vi "Rescript.vi"() -> ()   [LabVIEW 2020]
uses:
  _Rescript/_Rescript/_Rescript.lvclass
  _Shared/_Shared.lvlib
  _Shared/Name Specs/Name Specs.lvclass
  _Shared/Tree/Tree.lvlib
panel:
  out "Target":string
  in  "Tree":string(tree)
  in  "OK":bool
  # "Disclaimer: Please consider committing changes before AND after this action."
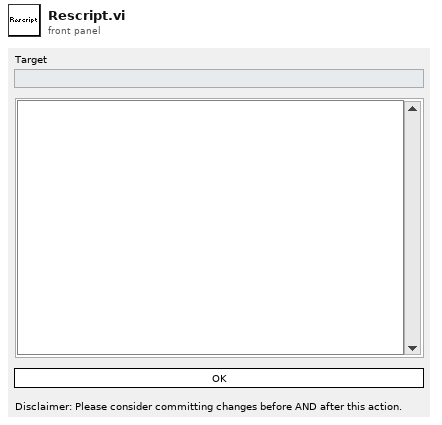
[diagram p1: front panel]
types:
  T1 = enum32{"Invalid", "Standard", "Closed", "Hidden", "Minimized", "Maximized"}
  T2 = typedef "_Shared.lvlib/Type Name Library File Path.ctl" = map{T3, T4}
  T3 = typedef "_Shared.lvlib/Type.ctl" = enum16{"Actor", "Msg"}
  T4 = typedef "_Shared.lvlib/Name Library File Path.ctl" = map{string, path}
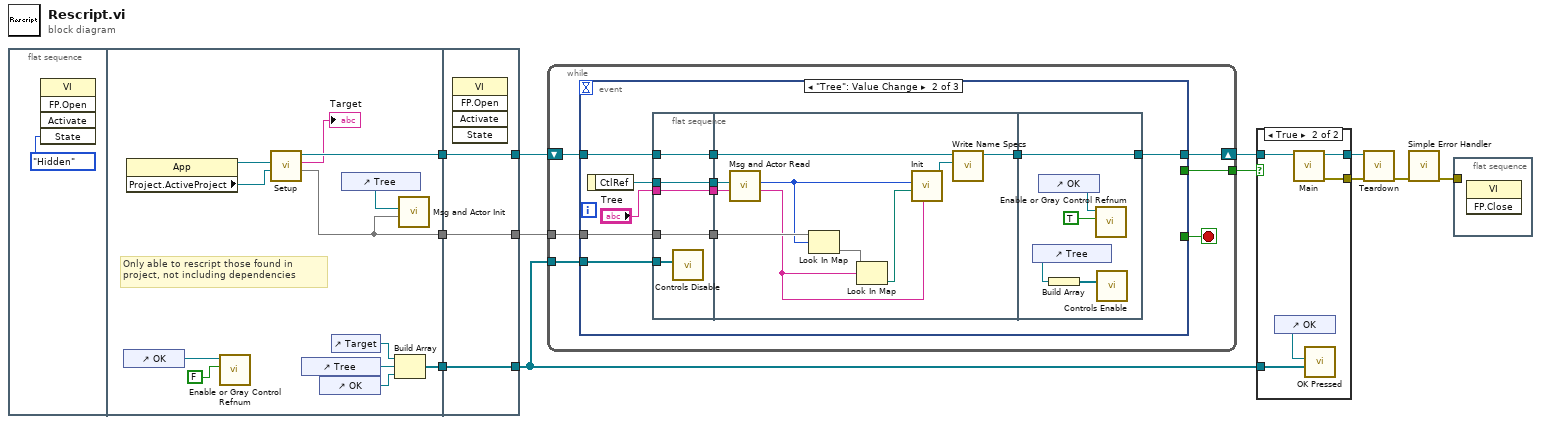
[diagram p0: block diagram]
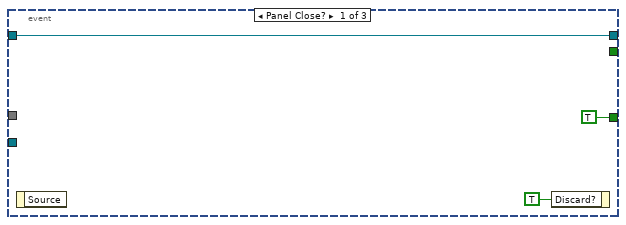
[diagram p2: hidden frame]
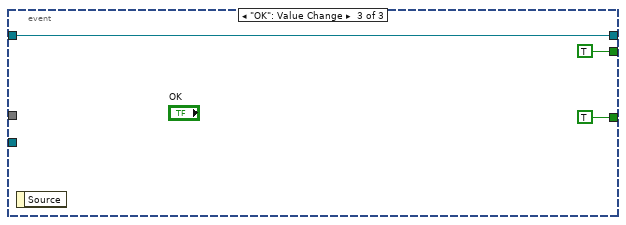
[diagram p3: hidden frame]
diagram:
  n1 = flat-sequence {
    tunnel: [w19] -> w8
    tunnel: [w14] -> w5
    tunnel: [w24] -> w4
    tunnel: [w28] -> w7
    tunnel: w8 -> [w28]
    tunnel: [w27] -> w6
    tunnel: w5 -> [w27]
    tunnel: [w26] -> w1
    tunnel: w4 -> [w26]
    frame #0 {
      n2 = invoke class="VI" method="FP.Open"("State"=T1."Hidden") -> ()  [unwired: 4 in, 5 out]
    }
    frame #1 {
      # "Only able to rescript those found in project, not including dependencies"
      n3 = control-ref of="OK"() -> (w23:refnum<vi>)
      n4 = property class="App"() -> (reference out=w20:refnum<vi>, "Project.ActiveProject"=w18:refnum<vi>)  [unwired: 2 in, 1 out]
      n5 = call <vilib>:"Enable or Gray Control Refnum.vi"("enable?"=FALSE, "Control in"=w23) -> ()  [unwired: 8 in, 2 out]
      n6 = call "Setup.vi"("Active Project"=w18, "NI.LV.Dialog Instance"=w20) -> ("Project Type Name Library File Path"=w14:T2, "Target"=→"Target":string, "_Rescript out"=w19:refnum<class "_Rescript.lvclass">)  [unwired: 6 in, 1 out]
      n7 = control-ref of="Tree"() -> (w21:refnum<vi>)
      n8 = control-ref of="OK"() -> (w25:refnum<vi>)
      n9 = control-ref of="Target"() -> (w16:refnum<vi>)
      n10 = control-ref of="Tree"() -> (w15:refnum<vi>)
      n11 = Build Array(w16, w21, w25) -> (w24:refnum<vi>[])
      n12 = call "Msg and Actor Init.vi"("Type Name Library File Path"=w14, "Tree Ref"=w15) -> ()  [unwired: 10 in]
    }
    frame #2 {
      n13 = invoke class="VI" method="FP.Open"() -> ()  [unwired: 5 in, 5 out]
    }
  }
  n14 = while {
    tunnel: [w34] -> w10
    shift-right: [w31] -> w9
    shift-left: w7 -> [w32]
    tunnel: w6 -> [w30]
    tunnel: w1 -> [w29]
    stop <- w33 stop-if-true
    n15 = event shown="[1] \"Tree\": Value Change" {
      selector: _ -> [_ _ _]
      dyn-events: _ -> [_ _ _]
      timeout: _ -> [_ _ _]
      tunnel: [_ _ TRUE ("Rename 2")] -> w34
      tunnel: [TRUE _ TRUE] -> w33
      tunnel: w32 -> [w35 w42 w71]
      tunnel: [w35 w48 w71] -> w31
      tunnel: w30 -> [_ w45 _]
      tunnel: w29 -> [_ w43 _]
      event Panel Close? {
        n16 = event-data() -> ()  [unwired: 1 in, 1 out]
        n17 = event-data("Discard?"=TRUE) -> ()  [unwired: 1 in, 1 out]
      }
      event "Tree": Value Change {
        n18 = event-data() -> ("CtlRef"=w40:refnum<vi>)  [unwired: 1 in]
        n19 = flat-sequence {
          tunnel: w42 -> [w53]
          tunnel: [w53] -> w46
          tunnel: w45 -> [w52]
          tunnel: [w52] -> w44
          tunnel: w43 -> [w51]
          tunnel: [w50] -> w41
          tunnel: w40 -> [w50]
          tunnel: "Tree" -> [w49]
          tunnel: [w49] -> w38
          tunnel: [w61] -> w47
          tunnel: w46 -> [w62]
          tunnel: w44 -> [w58]
          tunnel: w41 -> [w60]
          tunnel: w38 -> [w59]
          tunnel: [w68] -> w48
          tunnel: w47 -> [w68]
          frame #0 {
            n20 = call "Controls Disable.vi"("Controls in"=w51) -> ()  [unwired: 11 in]
          }
          frame #1 {
            n21 = call "Msg and Actor Read.vi"("Tree"=w59, "Tree Ref"=w60) -> ("Name"=w55:string, "Type"=w57:T3)  [unwired: 8 in]
            n22 = Look In Map(map=w58, key=w57) -> (value=w56:T4)  [unwired: 1 in, 1 out]
            n23 = Look In Map(map=w56, key=w55) -> (value=w54:path)  [unwired: 1 in, 1 out]
            n24 = call "Init.vi"("Name"=w55, "Name Library File Path"=w54, "Type"=w57) -> ("Name Specs out"=w63:refnum<class "Name Specs.lvclass">)  [unwired: 8 in]
            n25 = call "Write Name Specs.vi"("Name Specs"=w63, "Rescript in"=w62) -> ("_Rescript out"=w61:refnum<class "_Rescript.lvclass">)  [unwired: 9 in]
          }
          frame #2 {
            n26 = control-ref of="Tree"() -> (w64:refnum<vi>)
            n27 = control-ref of="OK"() -> (w67:refnum<vi>)
            n28 = Build Array(w64) -> (w65:refnum<vi>[])
            n29 = call <vilib>:"Enable or Gray Control Refnum.vi"("enable?"=TRUE, "Control in"=w67) -> ()  [unwired: 8 in, 2 out]
            n30 = call "Controls Enable.vi"("Controls in"=w65) -> ()  [unwired: 11 in]
          }
        }
      }
      event "OK": Value Change {
        n31 = event-data() -> ()  [unwired: 1 in, 1 out]
      }
    }
  }
  n32 = case shown="True" w10 {
    tunnel: w9 -> [w72 w77]
    tunnel: [w72 w76] -> w12
    tunnel: w1 -> [_ w74]
    tunnel: [_ w75] -> w11
    frame False {
    }
    frame True {
      n33 = control-ref of="OK"() -> (w73:refnum<vi>)
      n34 = call "Main.vi"("_Rescript in"=w77) -> ("error out"=w75:errorcluster, "_Rescript out"=w76:refnum<class "_Rescript.lvclass">)  [unwired: 9 in]
      n35 = call "OK Pressed.vi"("Controls in"=w74, "OK Ref"=w73) -> ()  [unwired: 10 in]
    }
  }
  n36 = call "Teardown.vi"("error in"=w11, "_Rescript in"=w12) -> ("error out"=w3:errorcluster)  [unwired: 9 in]
  n37 = call <vilib>:"Simple Error Handler.vi"("error in (no error)"=w3) -> ("error out"=w2:errorcluster)  [unwired: 4 in, 4 out]
  n38 = flat-sequence {
    tunnel: w2 -> [_]
    frame #0 {
      n39 = invoke class="VI" method="FP.Close"() -> ()  [unwired: 3 in, 3 out]
    }
  }
